vi "Read F4T .Net refnum.vi"(8 "error in (no error)":errorcluster, 11 "F4T in":refnum<class "F4T.lvclass">) -> (0 "error out":errorcluster, 2 "F4T .Net refnum":refnum<k24>, 3 "F4T out":refnum<class "F4T.lvclass">)   [LabVIEW 2018, in "F4T.lvlib" / "F4T.lvclass"]
uses:
  F4T.lvclass
  C:/Program Files/National Instruments/LabVIEW 2018/instr.lib/Watlow Std Bus/Public/Watbus.dll
  Program Files/National Instruments/LabVIEW 2018/instr.lib/Watlow Std Bus/Public/Watbus.dll
  F4T.lvclass/F4T.ctl
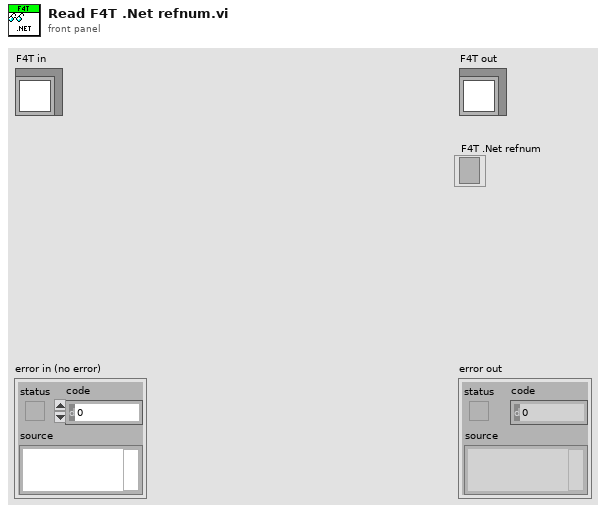
[diagram p1: front panel]
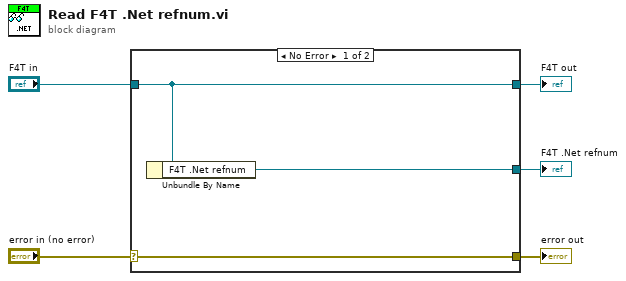
[diagram p0: block diagram]
diagram:
  n1 = case shown="No Error" "error in (no error)" {
    selector: "error in (no error)" -> [w8 w9]
    tunnel: [w8 w9] -> w4
    tunnel: [w7 w10] -> w2
    tunnel: "F4T in" -> [w7 w10]
    tunnel: [w6 _] -> w1
    frame No Error {
      n2 = Unbundle By Name(w7) -> ("F4T .Net refnum"=w6:refnum<k24>)
    }
    frame Error {
    }
  }
  "error out" <- w4
  "F4T out" <- w2
  "F4T .Net refnum" <- w1
